vi "Test.vi"() -> ()   [LabVIEW 2011]
uses:
  JSON GetSet.lvlib
  Variant JSON/Add Array of Variant to JSON Object.vi
  Variant JSON/Variant JSON.lvlib
  JSON Scalar/Get as EXT.vi
  JSON Scalar/JSON Scalar.lvclass
panel:
  out "Array of numbers":dbl[](array[numeric])
  out "Number":ext format="%.2f"
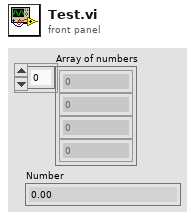
[diagram p1: front panel]
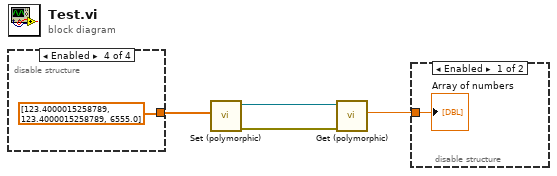
[diagram p0: block diagram]
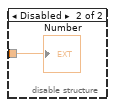
[diagram p2: hidden frame]
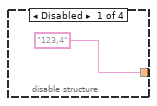
[diagram p3: hidden frame]
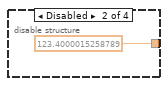
[diagram p4: hidden frame]
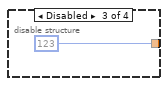
[diagram p5: hidden frame]
diagram:
  n1 = disable-structure shown="Enabled" {
    disable-tunnel: ["123,4" 123.4000015258789 123 dbl[] [123.4000015258789, 123.4000015258789, 6555.0]] -> w2
    frame Disabled {
    }
    frame Disabled {
    }
    frame Disabled {
    }
    frame Enabled {
    }
  }
  n2 = call-poly "Set (polymorphic).vi"("Array of Variants (with names)"=w2) -> ("error out"=w3:errorcluster, "JSON Object with items added"=w4:refnum<class "JSON Object.lvclass">)  [unwired: 9 in]
  n3 = call-poly "Get (polymorphic).vi"("error in (no error)"=w3, "JSON Value in"=w4) -> ("Number"=w1:ext)  [unwired: 7 in, 2 out]
  n4 = disable-structure shown="Enabled" {
    disable-tunnel: w1 -> [w9 w10]
    frame Enabled {
      "Array of numbers" <- w9
    }
    frame Disabled {
      "Number" <- w10
    }
  }
